vi "ConnectionStatus.vi"(11 "Connection Status":bool) -> (0 "String":string="Connections: Terminate\nConnections: Initialize", 3 "SystemStatus":bool)   [LabVIEW 2020]
panel:
  in  "Connect":bool
  out "Connection":bool
  in  "OK":bool
  # "System Connection"
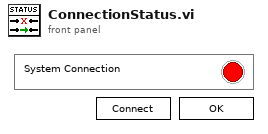
[diagram p1: front panel]
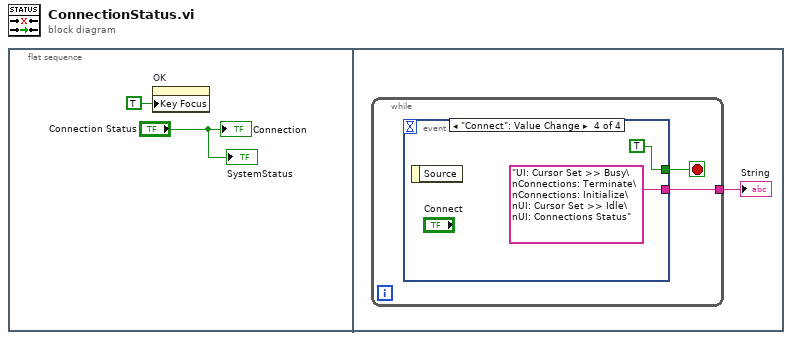
[diagram p0: block diagram]
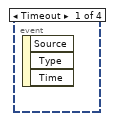
[diagram p2: hidden frame]
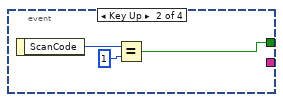
[diagram p3: hidden frame]
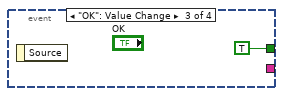
[diagram p4: hidden frame]
diagram:
  n1 = flat-sequence {
    frame #0 {
      n2 = property on="OK" class="Bool"("Key Focus"=TRUE) -> ()  [unwired: 2 in, 2 out]
      "Connection" <- "Connection Status"
      "SystemStatus" <- "Connection Status"
    }
    frame #1 {
      n3 = while {
        tunnel: [w4] -> w3
        stop <- w5 stop-if-true
        n4 = event shown="[3] \"Connect\": Value Change" {
          selector: _ -> [_ _ _ _]
          dyn-events: _ -> [_ _ _ _]
          timeout: _ -> [_ _ _ _]
          tunnel: [_ w6 TRUE TRUE] -> w5
          tunnel: [_ _ _ "UI: Cursor Set >> Busy\nConnections: Terminate\nConnections: Initialize\nUI: Cursor Set >> Idle\nUI: Connections Status"] -> w4
          event Timeout {
            n5 = event-data() -> ()  [unwired: 1 in, 3 out]
          }
          event Key Up {
            n6 = event-data() -> ("ScanCode"=w8:i16)  [unwired: 1 in]
            n7 = Equal?(x=w8, y=i16 1) -> (x = y?=w6:bool)
          }
          event "OK": Value Change {
            n8 = event-data() -> ()  [unwired: 1 in, 1 out]
          }
          event "Connect": Value Change {
            n9 = event-data() -> ()  [unwired: 1 in, 1 out]
          }
        }
      }
      "String" <- w3
    }
  }
